vi "string array.vi"(2 "String N":i32[](array[numeric]), 3 "Input String":string[](array[string])) -> (0 "Output String":string[](array[string]), 1 "after item":string[](array[string])=["Date time", "Shoe #", "Shoe Type", "Shoe Lv.", "Run time", "Step", "Distance (km)", "Earn GST", "Energy", "durability", "Δdura."])   [LabVIEW 2016]
panel:
  out "before item":string[](array[string])=["Run time & STEP", "Earn GST", "Energy", "Distance(km)", "Date time", "Shoe Type & Lv.", "Shoe #", "durability", "Δdura"]
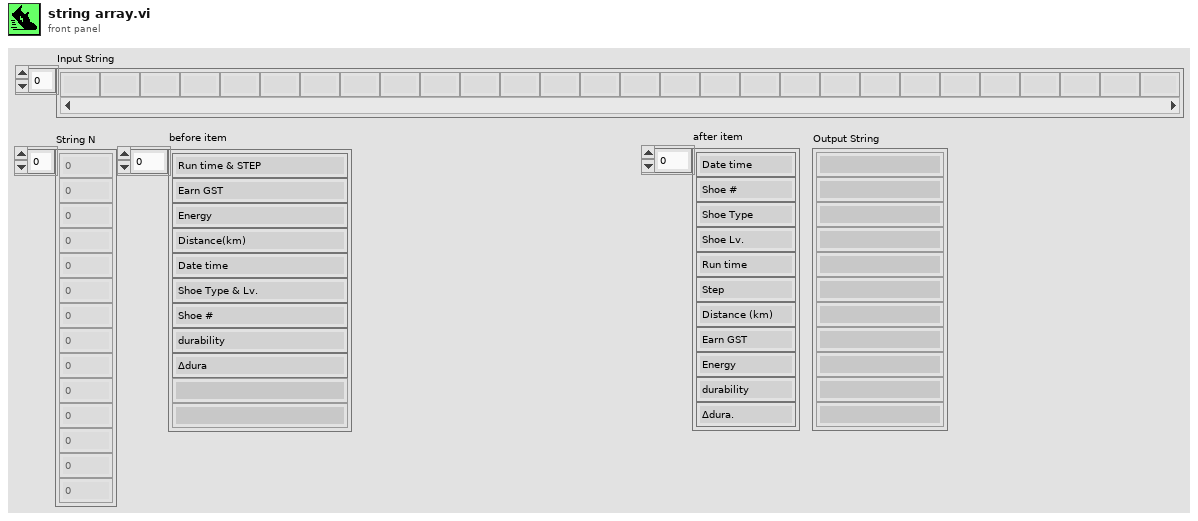
[diagram p1: front panel]
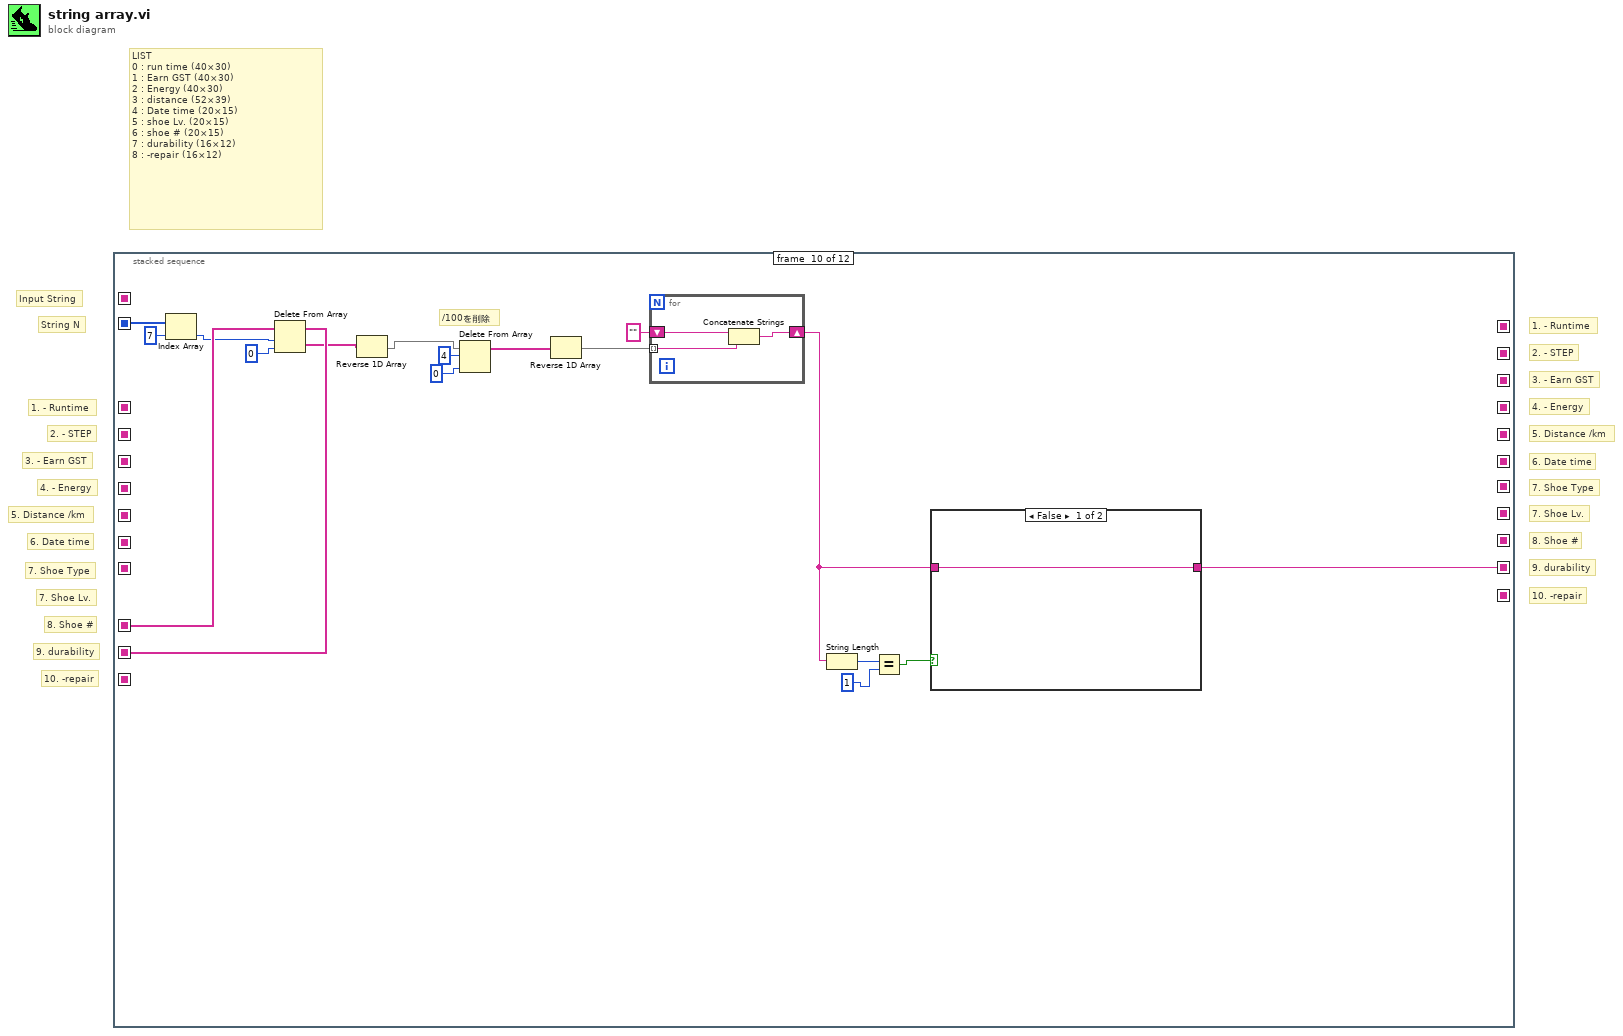
[diagram p0: block diagram]
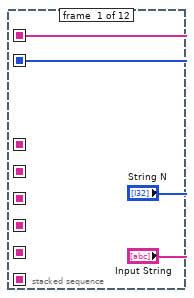
[diagram p2: hidden frame]
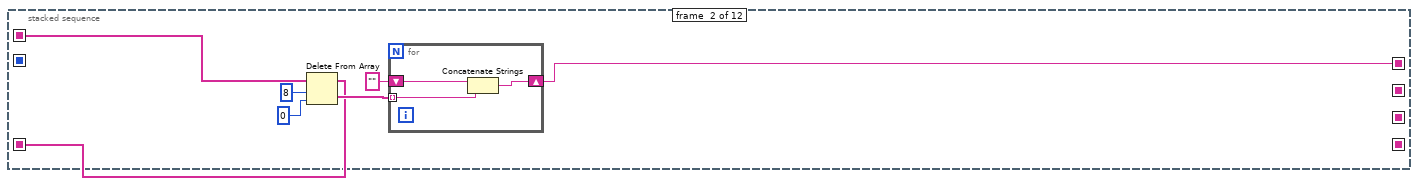
[diagram p3: hidden frame]
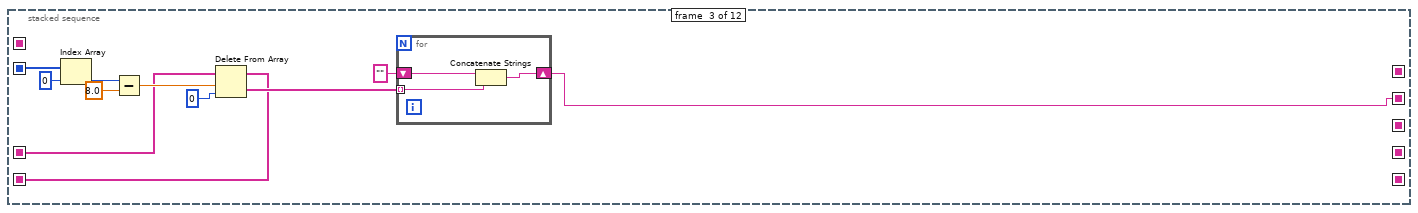
[diagram p4: hidden frame]
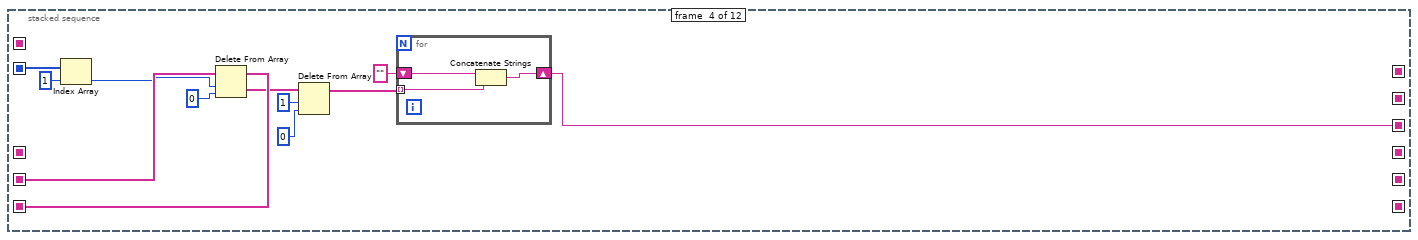
[diagram p5: hidden frame]
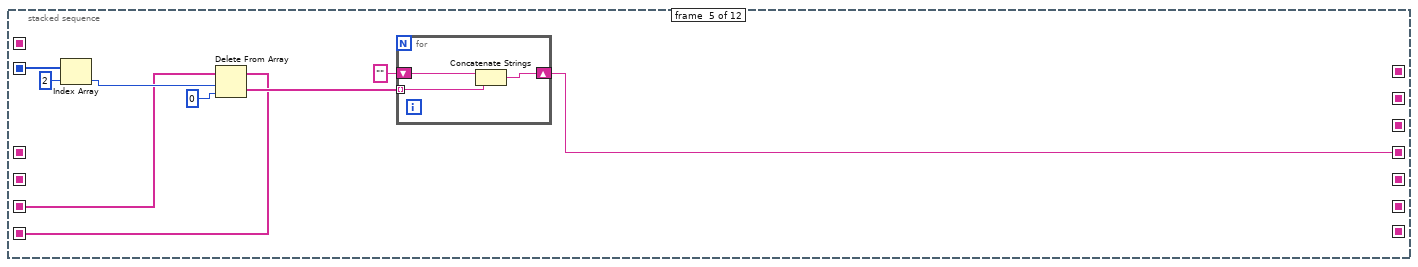
[diagram p6: hidden frame]
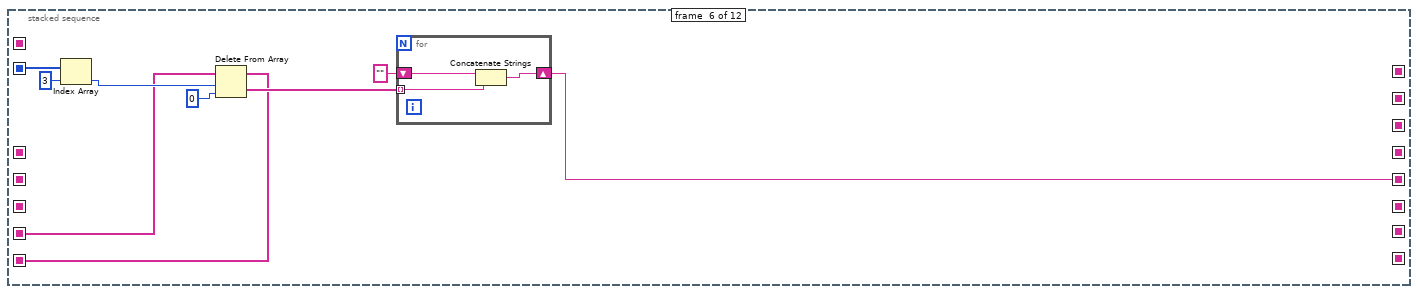
[diagram p7: hidden frame]
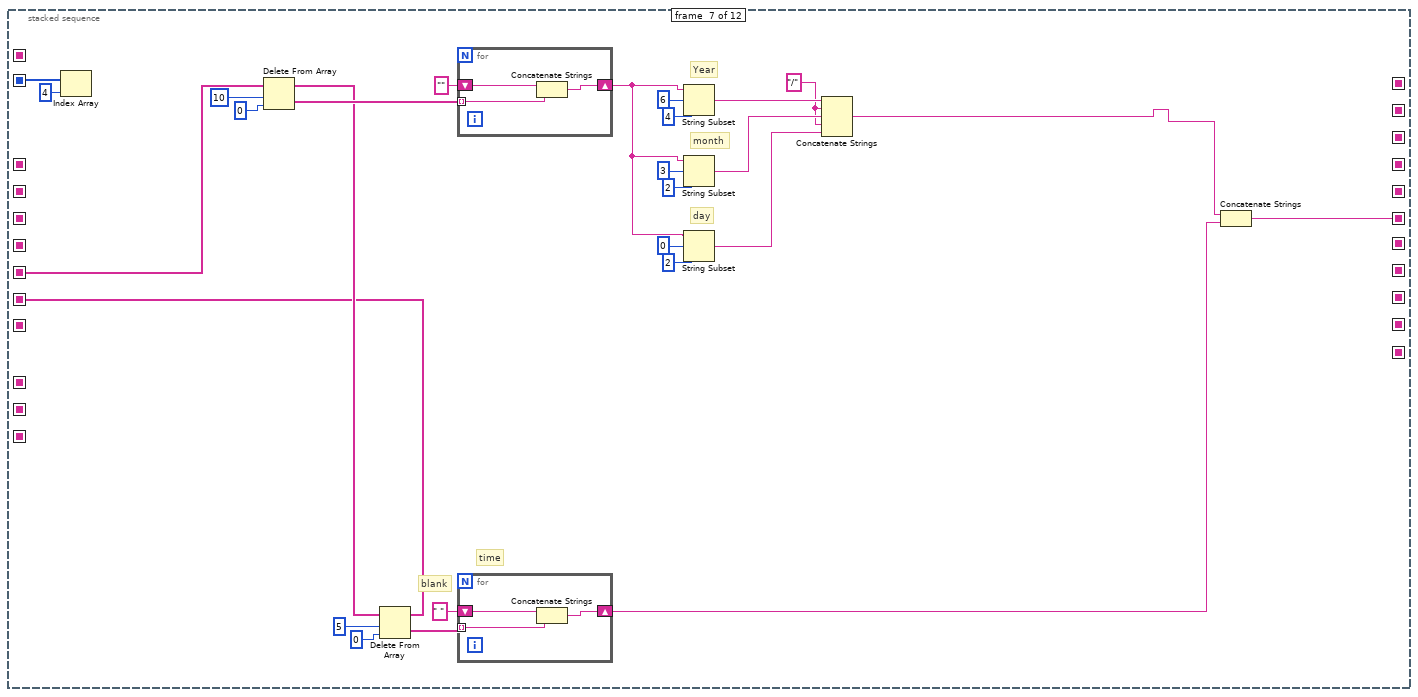
[diagram p8: hidden frame]
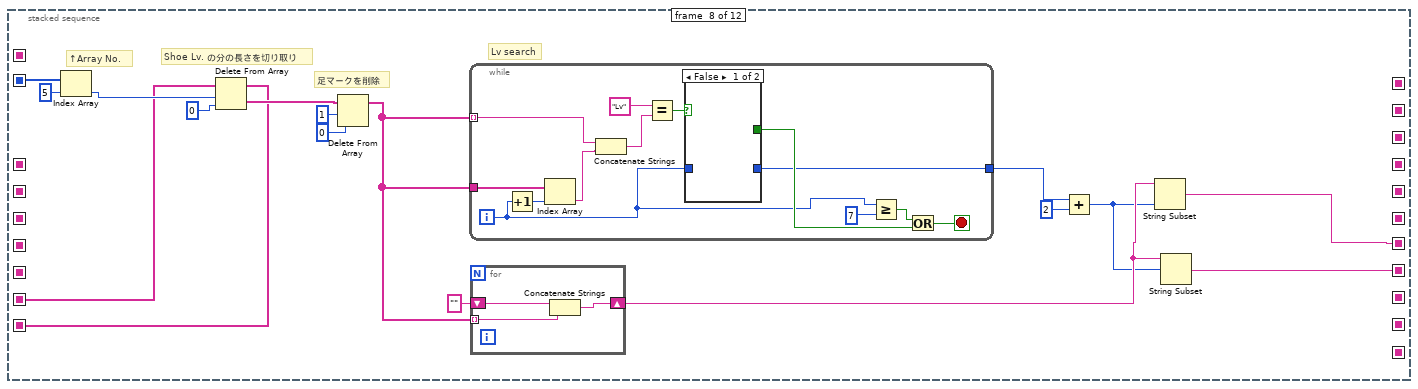
[diagram p9: hidden frame]
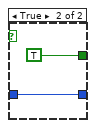
[diagram p10: hidden frame]
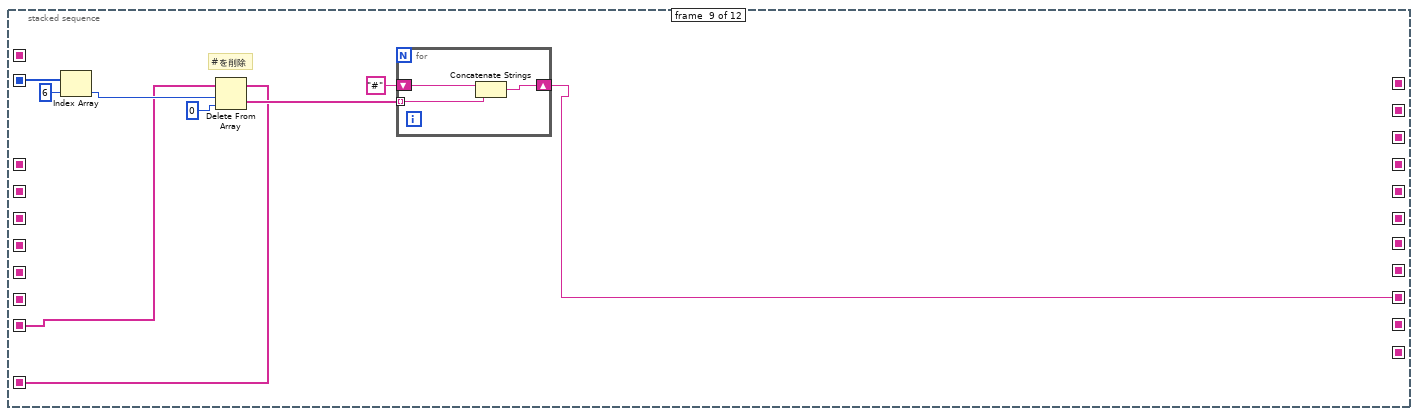
[diagram p11: hidden frame]
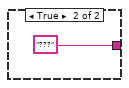
[diagram p12: hidden frame]
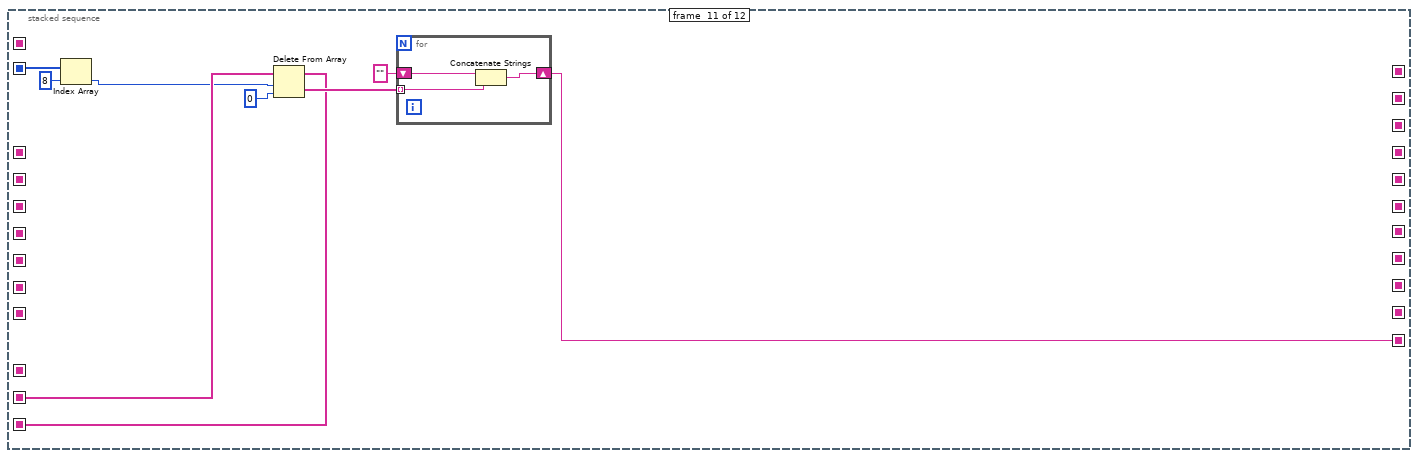
[diagram p13: hidden frame]
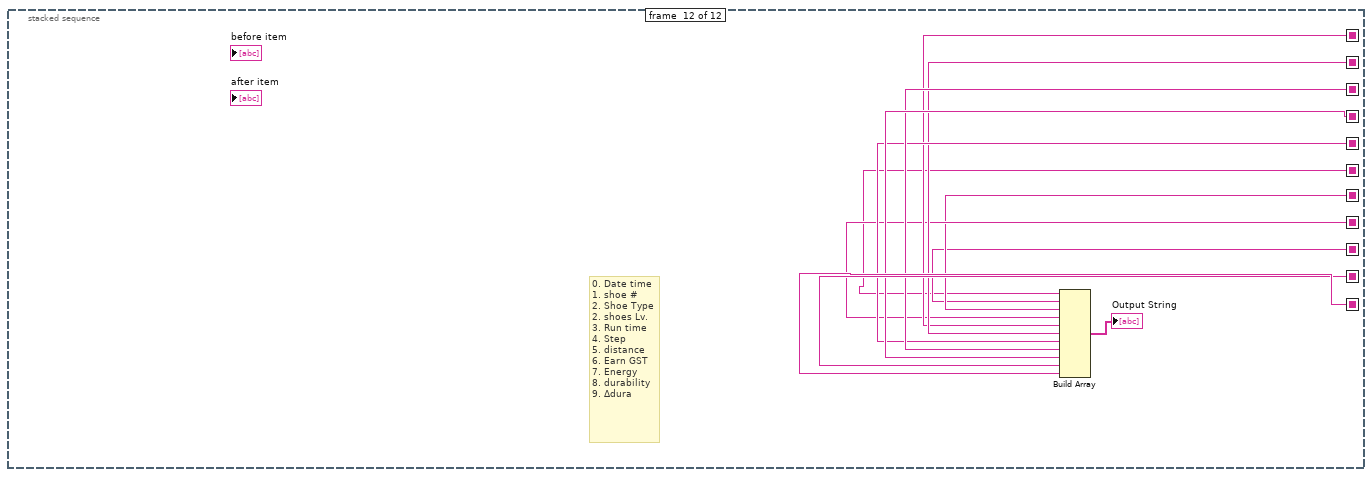
[diagram p14: hidden frame]
diagram:
  # "7. Shoe Type"
  # "7. Shoe Type"
  # "10. -repair"
  # "9. durability"
  # "8. Shoe #"
  # "7. Shoe Lv."
  # "6. Date time"
  # "5. Distance /km"
  # "4. - Energy"
  # "3. - Earn GST"
  # "2. - STEP"
  # "1. - Runtime"
  # "10. -repair"
  # "9. durability"
  # "8. Shoe #"
  # "7. Shoe Lv."
  # "6. Date time"
  # "5. Distance /km"
  # "LIST\n0 : run time (40×30)\n1 : Earn GST (40×30)\n2 : Energy (40×30)\n3 : distance (52×39)\n4 : Date time (20×15)\n5 : shoe Lv. (20×15)\n6 : shoe # (20×15)\n7 : durability (16×12)\n8 : -repair (16×12)"
  # "4. - Energy"
  # "3. - Earn GST"
  # "2. - STEP"
  # "1. - Runtime"
  # "String N"
  # "Input String"
  n1 = stacked-sequence {
    seq-local: ["Input String" _ _ _ _ _ _ _ _ _ _ _] -> [_ w5 _ _ _ _ _ _ _ _ _ _]
    seq-local: ["String N" _ _ _ _ _ _ _ _ _ _ _] -> [_ _ w17 w35 w46 w58 w88 w113 w138 w160 w173 _]
    seq-local: [_ w4 _ _ _ _ _ _ _ _ _ _] -> [_ _ w15 _ _ _ _ _ _ _ _ _]
    seq-local: [_ _ w14 _ _ _ _ _ _ _ _ _] -> [_ _ _ w34 _ _ _ _ _ _ _ _]
    seq-local: [_ _ _ w33 _ _ _ _ _ _ _ _] -> [_ _ _ _ w43 _ _ _ _ _ _ _]
    seq-local: [_ _ _ _ w44 _ _ _ _ _ _ _] -> [_ _ _ _ _ w56 _ _ _ _ _ _]
    seq-local: [_ _ _ _ _ w55 _ _ _ _ _ _] -> [_ _ _ _ _ _ w87 _ _ _ _ _]
    seq-local: [_ _ _ _ _ _ w81 _ _ _ _ _] -> [_ _ _ _ _ _ _ w111 _ _ _ _]
    seq-local: [_ _ _ _ _ _ _ _ w134 _ _ _] -> [_ _ _ _ _ _ _ _ _ w159 _ _]
    seq-local: [_ _ _ _ _ _ _ _ _ w155 _ _] -> [_ _ _ _ _ _ _ _ _ _ w171 _]
    seq-local: [_ _ _ _ _ _ _ _ _ _ w172 _] -> [_ _ _ _ _ _ _ _ _ _ _ _]
    seq-local: [_ w3 _ _ _ _ _ _ _ _ _ _] -> [_ _ _ _ _ _ _ _ _ _ _ w185]
    seq-local: [_ _ w13 _ _ _ _ _ _ _ _ _] -> [_ _ _ _ _ _ _ _ _ _ _ w186]
    seq-local: [_ _ _ w32 _ _ _ _ _ _ _ _] -> [_ _ _ _ _ _ _ _ _ _ _ w188]
    seq-local: [_ _ _ _ _ _ _ _ _ w146 _ _] -> [_ _ _ _ _ _ _ _ _ _ _ w190]
    seq-local: [_ _ _ _ _ _ _ _ _ _ w169 _] -> [_ _ _ _ _ _ _ _ _ _ _ w191]
    seq-local: [_ _ _ _ _ _ _ w100 _ _ _ _] -> [_ _ _ _ _ _ _ _ _ _ _ w184]
    seq-local: [_ _ _ _ _ _ _ _ w136 _ _ _] -> [_ _ _ _ _ _ _ _ _ _ _ w182]
    seq-local: [_ _ _ _ _ w54 _ _ _ _ _ _] -> [_ _ _ _ _ _ _ _ _ _ _ w187]
    seq-local: [_ _ _ _ _ _ w78 _ _ _ _ _] -> [_ _ _ _ _ _ _ _ _ _ _ w181]
    seq-local: [_ _ _ _ w42 _ _ _ _ _ _ _] -> [_ _ _ _ _ _ _ _ _ _ _ w189]
    seq-local: [_ _ _ _ _ _ _ w107 _ _ _ _] -> [_ _ _ _ _ _ _ _ w135 _ _ _]
    seq-local: [_ _ _ _ _ _ _ w99 _ _ _ _] -> [_ _ _ _ _ _ _ _ _ _ _ w183]
    frame #0 {
    }
    frame #1 {
      n2 = Delete From Array(array=w5, length=8, index=0 ("指標")) -> (deleted portion=w8:string[], array with subset deleted=w4:string[])
      n3 = for {
        tunnel: w8 -> [w10] mode=indexing
        shift-right: [w12] -> w3
        shift-left: "" -> [w11]
        n4 = Concatenate Strings(w11, w10) -> (w12:string)
      }
    }
    frame #2 {
      n5 = Index Array(array=w17, index=0 ("指標")) -> (element=w16:i32)
      n6 = Subtract(x=w16, y=8.0) -> (x-y=w21:dbl)
      n7 = Delete From Array(array=w15, length=w21, index=0 ("指標")) -> (deleted portion=w19:string[], array with subset deleted=w14:string[])
      n8 = for {
        tunnel: w19 -> [w24] mode=indexing
        shift-right: [w26] -> w13
        shift-left: "" -> [w25]
        n9 = Concatenate Strings(w25, w24) -> (w26:string)
      }
    }
    frame #3 {
      n10 = Index Array(array=w35, index=1 ("指標")) -> (element=w31:i32)
      n11 = Delete From Array(array=w34, length=w31, index=0 ("指標")) -> (deleted portion=w30:string[], array with subset deleted=w33:string[])
      n12 = Delete From Array(array=w30, length=1 ("長さ"), index=0 ("指標")) -> (array with subset deleted=w27:string[])  [unwired: 1 out]
      n13 = for {
        tunnel: w27 -> [w39] mode=indexing
        shift-right: [w41] -> w32
        shift-left: "" -> [w40]
        n14 = Concatenate Strings(w40, w39) -> (w41:string)
      }
    }
    frame #4 {
      n15 = Index Array(array=w46, index=2 ("指標")) -> (element=w45:i32)
      n16 = Delete From Array(array=w43, length=w45, index=0 ("指標")) -> (deleted portion=w47:string[], array with subset deleted=w44:string[])
      n17 = for {
        tunnel: w47 -> [w51] mode=indexing
        shift-right: [w53] -> w42
        shift-left: "" -> [w52]
        n18 = Concatenate Strings(w52, w51) -> (w53:string)
      }
    }
    frame #5 {
      n19 = Index Array(array=w58, index=3 ("指標")) -> (element=w57:i32)
      n20 = Delete From Array(array=w56, length=w57, index=0 ("指標")) -> (deleted portion=w59:string[], array with subset deleted=w55:string[])
      n21 = for {
        tunnel: w59 -> [w63] mode=indexing
        shift-right: [w65] -> w54
        shift-left: "" -> [w64]
        n22 = Concatenate Strings(w64, w63) -> (w65:string)
      }
    }
    frame #6 {
      w67 = "/"
      # "Year"
      # "month"
      # "day"
      # "time"
      # "blank"
      n23 = Index Array(array=w88, index=4 ("指標")) -> ()  [unwired: 1 out]
      n24 = Delete From Array(array=w87, length=10 ("y"), index=0 ("指標")) -> (deleted portion=w89:string[], array with subset deleted=w82:string[])
      n25 = Delete From Array(array=w82, length=5 ("y"), index=0 ("指標")) -> (deleted portion=w80:string[], array with subset deleted=w81:string[])
      n26 = for {
        tunnel: w89 -> [w96] mode=indexing
        shift-right: [w98] -> w71
        shift-left: "" -> [w97]
        n27 = Concatenate Strings(w97, w96) -> (w98:string)
      }
      n28 = for {
        tunnel: w80 -> [w93] mode=indexing
        shift-right: [w95] -> w79
        shift-left: " " -> [w94]
        n29 = Concatenate Strings(w94, w93) -> (w95:string)
      }
      n30 = String Subset(string=w71, offset (0)=6 ("長さ（残り）"), length (rest)=4 ("長さ（残り）")) -> (substring=w70:string)
      n31 = String Subset(string=w71, offset (0)=3 ("長さ（残り）"), length (rest)=2 ("長さ（残り）")) -> (substring=w69:string)
      n32 = String Subset(string=w71, offset (0)=0 ("長さ（残り）"), length (rest)=2 ("長さ（残り）")) -> (substring=w68:string)
      n33 = Concatenate Strings(w70, w67, w69, w67, w68) -> (w66:string)
      n34 = Concatenate Strings(w66, w79) -> (w78:string)
    }
    frame #7 {
      # "Lv search"
      # "足マークを削除"
      # "Shoe Lv. の分の長さを切り取り"
      # "↑Array No."
      n35 = Index Array(array=w113, index=5 ("指標")) -> (element=w112:i32)
      n36 = Delete From Array(array=w111, length=w112, index=0 ("指標")) -> (deleted portion=w108:string[], array with subset deleted=w107:string[])
      n37 = Delete From Array(array=w108, length=1 ("長さ"), index=0 ("指標")) -> (array with subset deleted=w105:string[])  [unwired: 1 out]
      n38 = while {
        tunnel: w105 -> [w124] mode=indexing
        tunnel: w105 -> [w127]
        tunnel: [w116] -> w104
        i -> [w117]
        stop <- w121 stop-if-true
        n39 = Increment(x=w117) -> (x+1=w126:i32)
        n40 = Index Array(array=w127, index=w126) -> (element=w123:string)
        n41 = Concatenate Strings(w124, w123) -> (w122:string)
        n42 = Equal?(x="Lv" ("検索文字列"), y=w122) -> (x = y?=w128:bool)
        n43 = case shown="False" w128 {
          tunnel: [_ TRUE] -> w120
          tunnel: w117 -> [_ w129]
          tunnel: [_ w129] -> w116
          frame False {
          }
          frame True {
          }
        }
        n44 = Greater Or Equal?(x=w117, y=7) -> (x >= y?=w118:bool)
        n45 = Or(x=w118, y=w120) -> (x .or. y?=w121:bool)
      }
      n46 = for {
        tunnel: w105 -> [w131] mode=indexing
        shift-right: [w133] -> w102
        shift-left: "" -> [w132]
        n47 = Concatenate Strings(w132, w131) -> (w133:string)
      }
      n48 = Add(x=w104, y=2) -> (x+y=w101:i32)
      n49 = String Subset(string=w102, length (rest)=w101) -> (substring=w99:string)  [unwired: 1 in]
      n50 = String Subset(string=w102, offset (0)=w101) -> (substring=w100:string)  [unwired: 1 in]
    }
    frame #8 {
      # "#を削除"
      n51 = Index Array(array=w138, index=6 ("指標")) -> (element=w137:i32)
      n52 = Delete From Array(array=w135, length=w137, index=0 ("指標")) -> (deleted portion=w139:string[], array with subset deleted=w134:string[])
      n53 = for {
        tunnel: w139 -> [w143] mode=indexing
        shift-right: [w145] -> w136
        shift-left: "#" -> [w144]
        n54 = Concatenate Strings(w144, w143) -> (w145:string)
      }
    }
    frame #9 {
      # "/100を削除"
      n55 = Index Array(array=w160, index=7 ("指標")) -> (element=w158:i32)
      n56 = Delete From Array(array=w159, length=w158, index=0 ("指標")) -> (deleted portion=w154:string[], array with subset deleted=w155:string[])
      n57 = Reverse 1D Array(array=w154) -> (reversed array=w153:string[])
      n58 = Delete From Array(array=w153, length=4 ("長さ"), index=0 ("指標")) -> (array with subset deleted=w151:string[])  [unwired: 1 out]
      n59 = Reverse 1D Array(array=w151) -> (reversed array=w152:string[])
      n60 = for {
        tunnel: w152 -> [w166] mode=indexing
        shift-right: [w168] -> w147
        shift-left: "" -> [w167]
        n61 = Concatenate Strings(w167, w166) -> (w168:string)
      }
      n62 = String Length(string=w147) -> (length=w150:i32)
      n63 = Equal?(x=w150, y=1 ("長さ")) -> (x = y?=w148:bool)
      n64 = case shown="False" w148 {
        tunnel: w147 -> [w164 _]
        tunnel: [w164 "???"] -> w146
        frame False {
        }
        frame True {
        }
      }
    }
    frame #10 {
      n65 = Index Array(array=w173, index=8 ("指標")) -> (element=w170:i32)
      n66 = Delete From Array(array=w171, length=w170, index=0 ("指標")) -> (deleted portion=w174:string[], array with subset deleted=w172:string[])
      n67 = for {
        tunnel: w174 -> [w178] mode=indexing
        shift-right: [w180] -> w169
        shift-left: "" -> [w179]
        n68 = Concatenate Strings(w179, w178) -> (w180:string)
      }
    }
    frame #11 {
      # "0. Date time\n1. shoe #\n2. Shoe Type\n2. shoes Lv.\n3. Run time\n4. Step\n5. distance\n6. Earn GST\n7. Energy\n8. durability\n9. Δdura"
      n69 = Build Array(w181, w182, w183, w184, w185, w186, w187, w188, w189, w190, w191) -> (→"Output String":string[])
    }
  }
